vi "Log String.vi"(6 "String":string, 8 "error in (no error)":errorcluster, 11 "Text File Sink in":refnum<class "Text File Sink.lvclass">) -> (0 "error out":errorcluster, 3 "Text File Sink out":refnum<class "Text File Sink.lvclass">)   [LabVIEW 2016, in "Stream Log.lvlib" / "Text File Sink.lvclass"]
doc: "--\nCopyright © 2017 Composed SystemsI All rights reserved.\n\nAuthor: Jon McBee <jon.mcbee@composed.io>\n\nThis library is provided \"AS IS\" ,WITHOUT WARRANTIES OR\nCONDITIONS OF ANY KIND, either express or implied.\n\nComposed Systems -- composed.io\n\nStream 0.0.1.1\nJon McBee - Composed Systems\nCopyright (c) 2017, Composed Systems"
uses:
  <userlib>/Composed Systems/Stream/Log/Text File Sink/Text File Sink.lvclass
  <userlib>/Composed Systems/Stream/Log/Text File Sink/Text File Sink.lvclass/Text File Sink.ctl
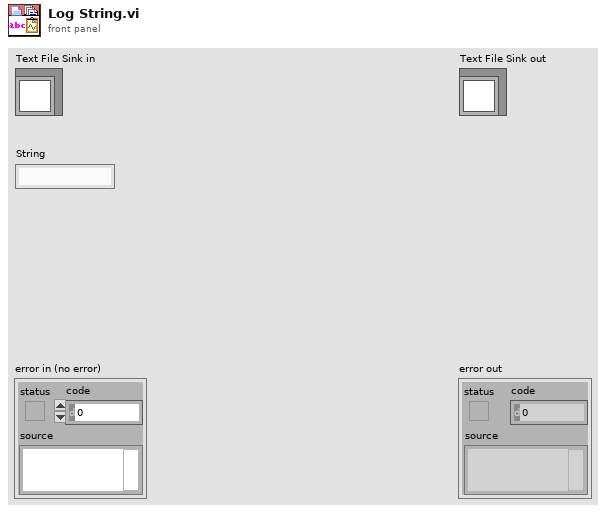
[diagram p1: front panel]
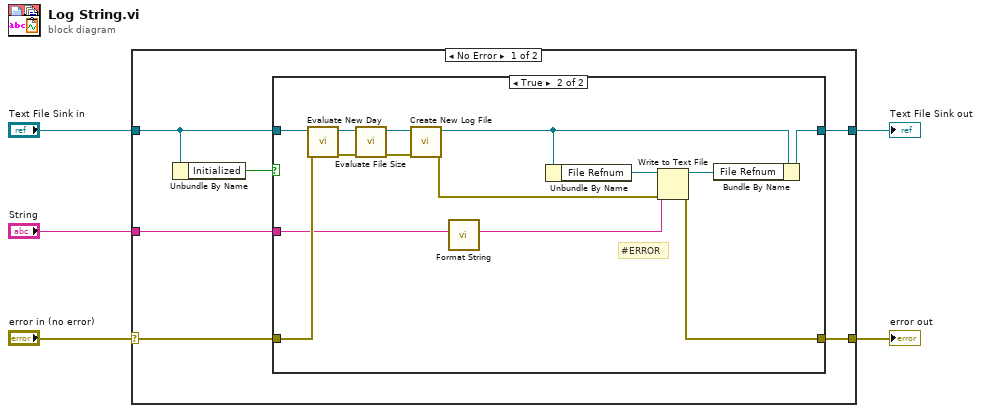
[diagram p0: block diagram]
diagram:
  n1 = case shown="No Error" "error in (no error)" {
    selector: "error in (no error)" -> [w10 w29]
    tunnel: [w9 w29] -> w4
    tunnel: "Text File Sink in" -> [w7 w28]
    tunnel: "String" -> [w8 _]
    tunnel: [w6 w28] -> w1
    frame No Error {
      n2 = Unbundle By Name(w7) -> ("Initialized"=w11:bool)
      n3 = case shown="True" w11 {
        tunnel: [w13 w16] -> w9
        tunnel: w10 -> [w13 w17]
        tunnel: w8 -> [_ w15]
        tunnel: w7 -> [w12 w27]
        tunnel: [w12 w22] -> w6
        frame False {
        }
        frame True {
          # "#ERROR"
          n4 = call <userlib>:"Evaluate New Day.vi"("error in (no error)"=w17, "Text File Sink in"=w27) -> ("error out"=w20:errorcluster, "Text File Sink out"=w26:refnum<class "Text File Sink.lvclass">)  [unwired: 8 in]
          n5 = call <userlib>:"Evaluate File Size.vi"("error in (no error)"=w20, "Text File Sink in"=w26) -> ("error out"=w19:errorcluster, "Text File Sink out"=w25:refnum<class "Text File Sink.lvclass">)  [unwired: 8 in]
          n6 = call <userlib>:"Create New Log File.vi"("error in (no error)"=w19, "Text File Sink in"=w25) -> ("error out"=w18:errorcluster, "Text File Sink out"=w23:refnum<class "Text File Sink.lvclass">)  [unwired: 8 in]
          n7 = call <userlib>:"Format String.vi"("String"=w15) -> ("Formatted String"=w14:string)  [unwired: 10 in]
          n8 = Unbundle By Name(w23) -> ("File Refnum"=w24:refnum<file>)
          n9 = Write to Text File(file (use dialog)=w24, text=w14, error in=w18) -> (refnum out=w21:refnum<file>, error out=w16:errorcluster)  [unwired: 2 out]
          n10 = Bundle By Name(cluster=w23, "File Refnum"=w21) -> (w22:refnum<class "Text File Sink.lvclass">)
        }
      }
    }
    frame Error {
    }
  }
  "error out" <- w4
  "Text File Sink out" <- w1
